vi "电源管理UI.vi"() -> ()   [LabVIEW 2016, in "PLC.lvlib"]
uses:
  PLC.lvlib
  <vilib>/Utility/miscctls.llb/LVPointTypeDef.ctl
  API/CodCr/CodCr.lvlib
panel:
  out "CODCr空闲时间":dbl caption="空闲时间:"
  out "总磷总氮空闲时间":dbl caption="空闲时间:"
  out "营养盐空闲时间":dbl caption="空闲时间:"
  out "CODMn空闲时间":dbl caption="空闲时间:"
  out "多参数空闲时间":dbl caption="空闲时间:"
  in  "CODCr电源":bool
  in  "总磷总氮电源":bool
  in  "营养盐电源":bool
  in  "CODMn电源":bool
  in  "多参数电源":bool
  # "说明：\n系统模式处于维护模式时，仪器电源自动打开；\n系统模式处于常规模式/质控模式/应急模式下，周期启动时，仪器电源打开，仪器空闲超过3600秒自动断电；"
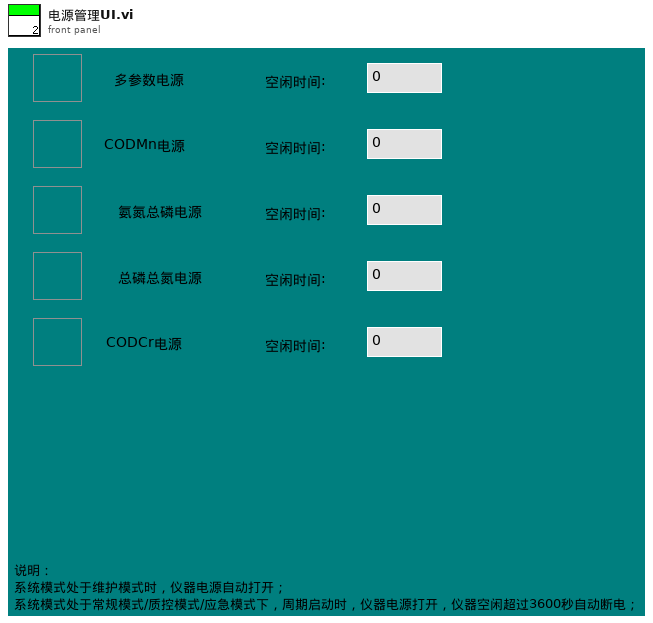
[diagram p1: front panel]
types:
  T1 = typedef "LVPointTypeDef.ctl" = cluster{"Horizontal":i16, "Vertical":i16}
  T2 = enum16{"空闲", "水样测试", "标样核查", "零点核查", "跨度核查", "空白测试", "平行样测试", "加标回收", "空白校准", "标样校准", "初始化（清洗）"}
  T3 = cluster{"系统时间":timestamp, "工作状态":u16, "测量模式":u16, "告警代码":enum16{"无告警", "缺试剂告警", "缺水样告警", "缺蒸馏水告警", "缺标液告警", "仪表漏液告警", "标定异常告警", "超量程告警", "加热异常", "低试剂预警", "超上限告警", "超下限告警", "仪表内部其他异常", "滴定异常告警", "电极异常告警", "量程切换告警", "参数设置告警", "PH电极电位异常", "电导率电极异常", "浊度光度异常", "溶解氧电极异常", "溶解氧光强异常", "温度异常告警", "PH异常告警", "溶解氧异常告警", "电导率异常告警", "浊度异常告警", "叶绿素异常告警", "藻密度异常告警", "蓝绿藻异常告警", "ORP异常告警", "氨氮异常告警", "清洁刷异常告警", "SD卡异常告警", "蓝牙异常告警", "Wifi异常告警", "流程异常告警"}, "故障代码":enum16{"无故障", "电机故障", "温度故障", "通讯故障", "滴定故障"}, "日志代码":u16, "软件版本":string}
  T4 = cluster{"系统时间":timestamp, "工作状态":enum16{"空闲", "水样测试", "标样核查", "零点核查", "跨度核查", "空白测试", "平行样测试", "加标回收", "空白校准", "标样校准", "初始化（清洗）"}, "测量模式":enum16{"待机", "连续模式", "周期模式", "定点模式", "受控模式", "手动模式"}, "告警代码":enum16{"无告警", "缺试剂告警", "缺水样告警", "缺蒸馏水告警", "缺标液告警", "仪表漏液告警", "标定异常告警", "超量程告警", "加热异常", "低试剂预警", "超上限告警", "超下限告警", "仪表内部其他异常", "滴定异常告警", "电极异常告警", "量程切换告警", "参数设置告警", "PH电极电位异常", "电导率电极异常", "浊度光度异常", "溶解氧电极异常", "溶解氧光强异常", "温度异常告警", "PH异常告警", "溶解氧异常告警", "电导率异常告警", "浊度异常告警", "叶绿素异常告警", "藻密度异常告警", "蓝绿藻异常告警", "ORP异常告警", "氨氮异常告警", "清洁刷异常告警", "SD卡异常告警", "蓝牙异常告警", "Wifi异常告警", "流程异常告警"}, "故障代码":enum16{"无故障", "电机故障", "温度故障", "通讯故障", "滴定故障"}, "日志代码":u16, "软件版本":u16, "F0":sgl, "F1":sgl, "F2":sgl, "F3":sgl, "T":sgl, "H":sgl, "id":u16, "flowid":u16, "量程":u16, "总磷控温温度1":sgl, "营养盐控温温度2":sgl, "ADC":sgl}
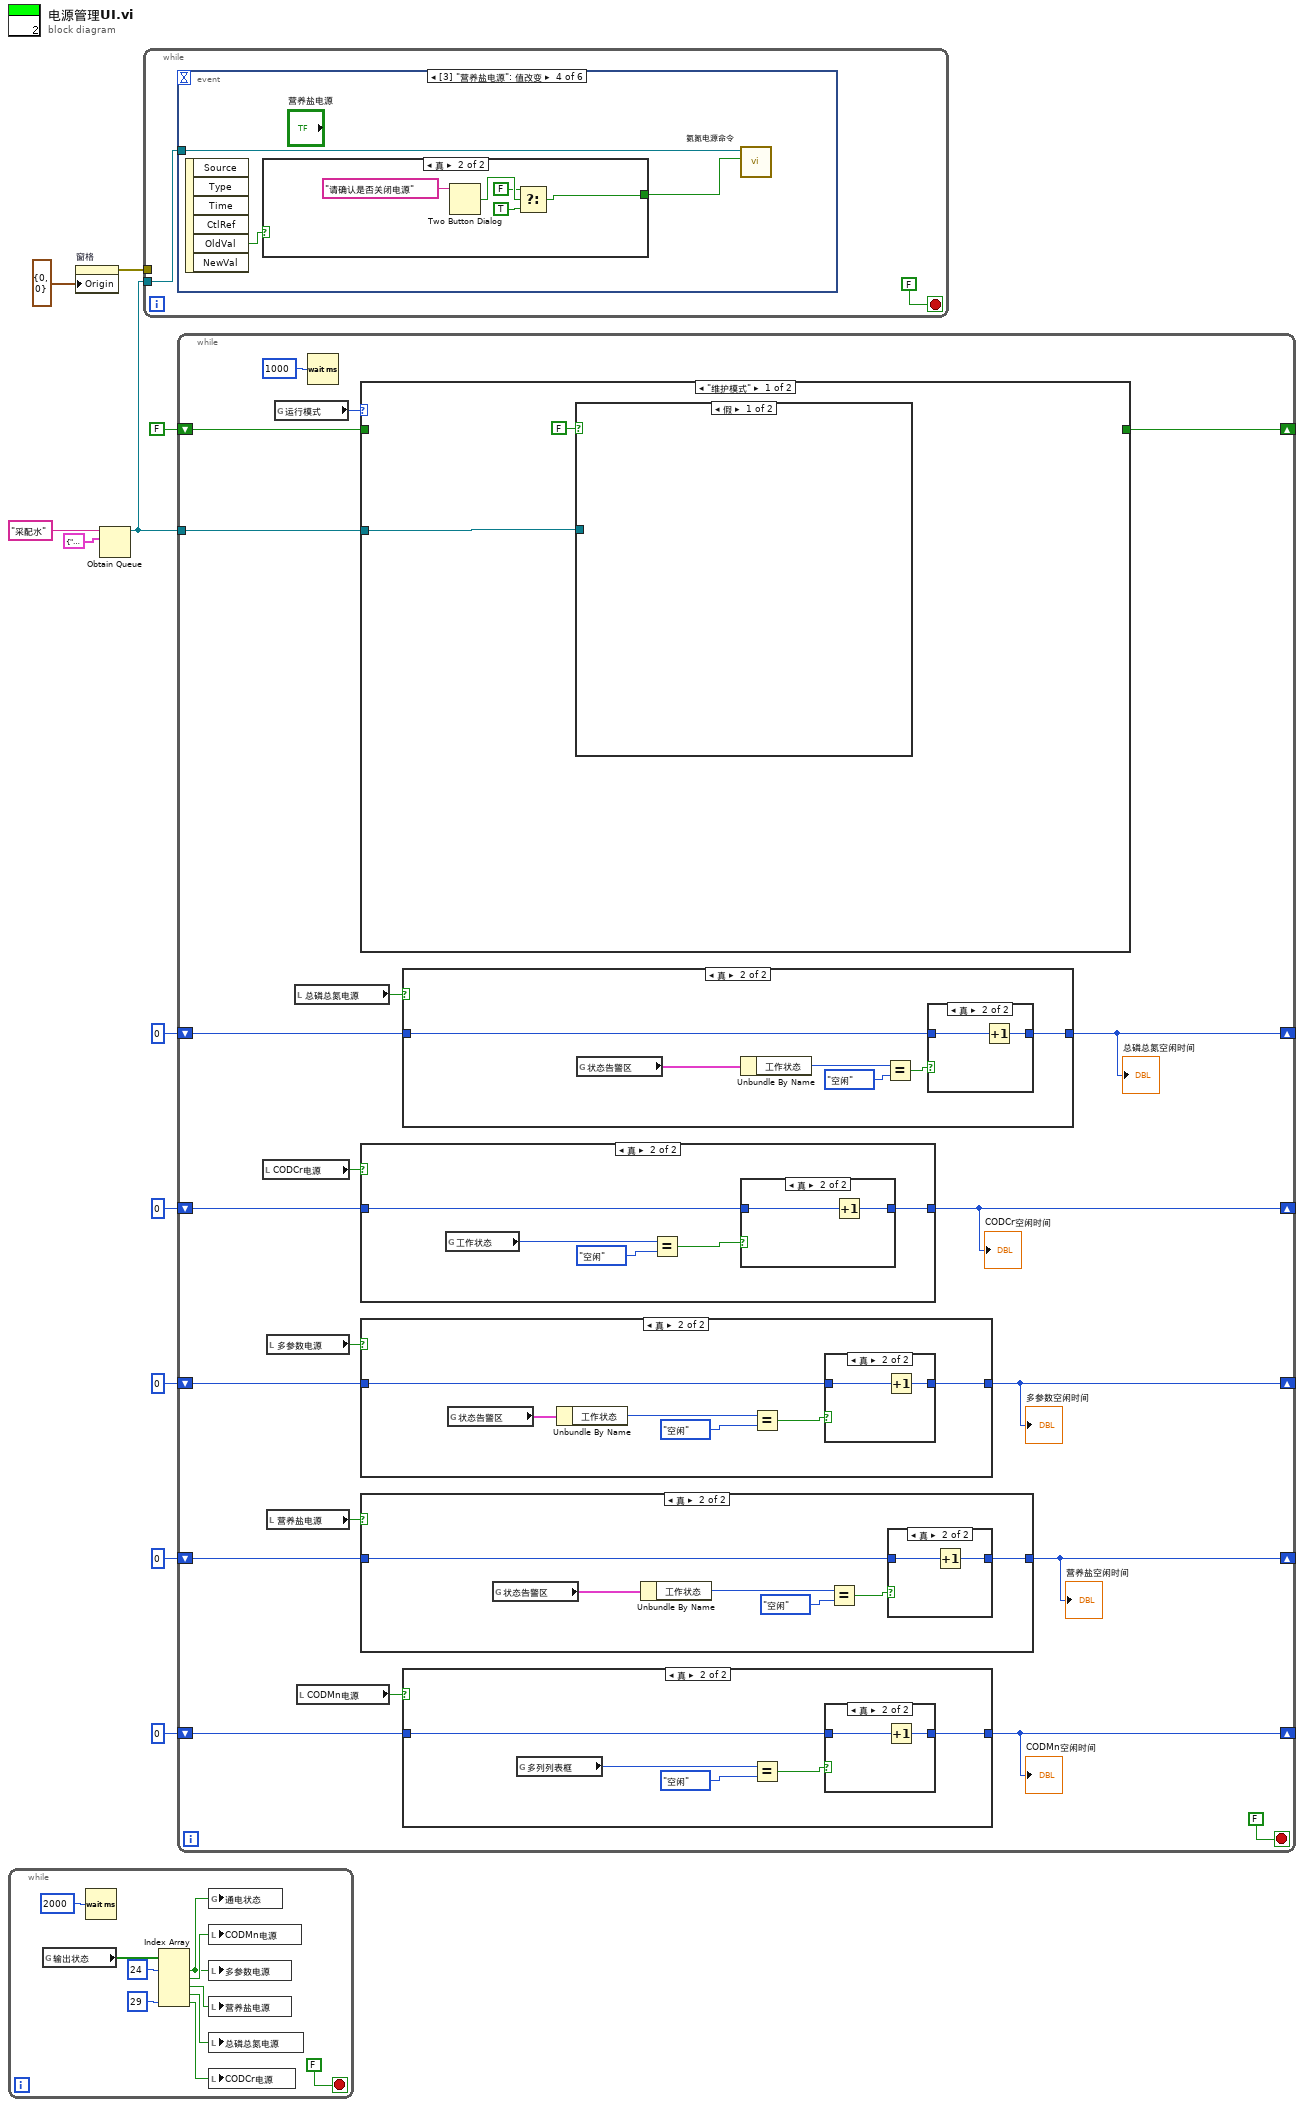
[diagram p0: block diagram]
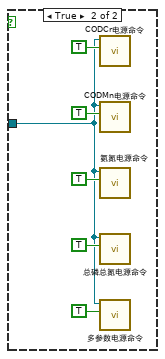
[diagram p2: hidden frame]
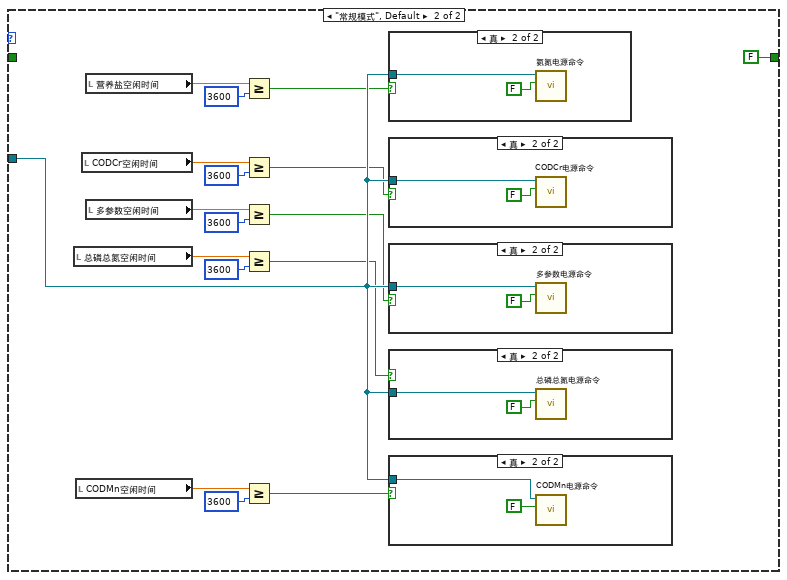
[diagram p3: hidden frame]
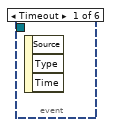
[diagram p19: hidden frame]
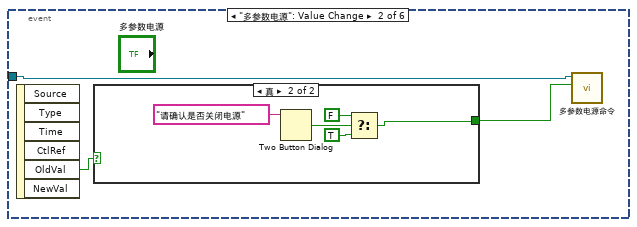
[diagram p20: hidden frame]
diagram:
  n1 = while {
    stop <- FALSE stop-if-true
    n2 = global read "采配水全局变量.vi" "输出状态"() -> (w19:bool[])
    n3 = Wait (ms)(milliseconds to wait=u32 2000 ("等待时间（毫秒）")) -> ()  [unwired: 1 out]
    n4 = Index Array(array=w19, index #1=24 ("索引"), index #5=29 ("索引")) -> (element #1=w14:bool, element #2=w17:bool, element #3=w16:bool, element #4=w15:bool, element #5=w13:bool)  [unwired: 3 in]
    n5 = global write "多参数全局变量.vi" "通电状态"(w14) -> ()
    n6 = local write "CODMn电源"(w17) -> ()
    n7 = local write "多参数电源"(w14) -> ()
    n8 = local write "营养盐电源"(w16) -> ()
    n9 = local write "总磷总氮电源"(w15) -> ()
    n10 = local write "CODCr电源"(w13) -> ()
  }
  n11 = property on="窗格" class="Pane"("Origin"=T1 {"Horizontal"=0, "Vertical"=0} ("原点")) -> (error out=w8:errorcluster)  [unwired: 2 in, 1 out]
  n12 = Obtain Queue(name (unnamed)="采配水" ("名称（未命名）"), element data type=cluster{"命令":string, "数据":variant} {"命令"="", "数据"=variant}) -> (queue out=w7:refnum<queue>)  [unwired: 3 in, 2 out]
  n13 = while {
    tunnel: w7 -> [w22]
    tunnel: w8 -> [_]
    stop <- FALSE stop-if-true
    n14 = event shown="[3] \"营养盐电源\": 值改变" {
      selector: _ -> [_ _ _ _ _ _]
      dyn-events: _ -> [_ _ _ _ _ _]
      timeout: _ -> [_ _ _ _ _ _]
      tunnel: w22 -> [_ w26 w35 w44 w53 w62]
      event Timeout {
        n15 = event-data() -> ()  [unwired: 1 in, 3 out]
      }
      event "多参数电源": Value Change {
        n16 = event-data() -> ("OldVal"=w25:bool)  [unwired: 1 in, 5 out]
        n17 = case shown="真" w25 {
          tunnel: [TRUE ("T button?") w28] -> w24
          frame False {
          }
          frame True {
            n18 = Two Button Dialog(message="请确认是否关闭电源" ("消息")) -> (T button?=w31:bool)  [unwired: 2 in]
            n19 = Select(t=FALSE, s=w31, f=TRUE ("T button?")) -> (s? t:f=w28:bool)
          }
        }
        n20 = call "多参数电源命令.vi"("通电/断电"=w24, "队列"=w26) -> ()  [unwired: 9 in, 1 out]
      }
      event "CODMn电源": Value Change {
        n21 = event-data() -> ("OldVal"=w34:bool)  [unwired: 1 in, 5 out]
        n22 = case shown="真" w34 {
          tunnel: [TRUE ("T button?") w37] -> w33
          frame False {
          }
          frame True {
            n23 = Two Button Dialog(message="请确认是否关闭电源" ("消息")) -> (T button?=w40:bool)  [unwired: 2 in]
            n24 = Select(t=FALSE, s=w40, f=TRUE ("T button?")) -> (s? t:f=w37:bool)
          }
        }
        n25 = call "CODMn电源命令.vi"("通电/断电"=w33, "队列"=w35) -> ()  [unwired: 9 in, 1 out]
      }
      event "营养盐电源": Value Change {
        n26 = event-data() -> ("OldVal"=w43:bool)  [unwired: 1 in, 5 out]
        n27 = case shown="真" w43 {
          tunnel: [TRUE ("T button?") w46] -> w42
          frame False {
          }
          frame True {
            n28 = Two Button Dialog(message="请确认是否关闭电源" ("消息")) -> (T button?=w49:bool)  [unwired: 2 in]
            n29 = Select(t=FALSE, s=w49, f=TRUE ("T button?")) -> (s? t:f=w46:bool)
          }
        }
        n30 = call "氨氮电源命令.vi"("通电/断电"=w42, "队列"=w44) -> ()  [unwired: 9 in, 1 out]
      }
      event "总磷总氮电源": Value Change {
        n31 = event-data() -> ("OldVal"=w52:bool)  [unwired: 1 in, 5 out]
        n32 = case shown="真" w52 {
          tunnel: [TRUE ("T button?") w55] -> w51
          frame False {
          }
          frame True {
            n33 = Two Button Dialog(message="请确认是否关闭电源" ("消息")) -> (T button?=w58:bool)  [unwired: 2 in]
            n34 = Select(t=FALSE, s=w58, f=TRUE ("T button?")) -> (s? t:f=w55:bool)
          }
        }
        n35 = call "总磷总氮电源命令.vi"("通电/断电"=w51, "队列"=w53) -> ()  [unwired: 9 in, 1 out]
      }
      event "CODCr电源": Value Change {
        n36 = event-data() -> ("OldVal"=w61:bool)  [unwired: 1 in, 5 out]
        n37 = case shown="真" w61 {
          tunnel: [TRUE ("T button?") w64] -> w60
          frame False {
          }
          frame True {
            n38 = Two Button Dialog(message="请确认是否关闭电源" ("消息")) -> (T button?=w67:bool)  [unwired: 2 in]
            n39 = Select(t=FALSE, s=w67, f=TRUE ("T button?")) -> (s? t:f=w64:bool)
          }
        }
        n40 = call "CODCr电源命令.vi"("通电/断电"=w60, "队列"=w62) -> ()  [unwired: 9 in, 1 out]
      }
    }
  }
  n41 = while {
    tunnel: w7 -> [w72]
    shift-right: [w73] -> _
    shift-left: u32 0 ("等待时间（毫秒）") -> [w86]
    shift-right: [w77] -> _
    shift-left: u32 0 ("等待时间（毫秒）") -> [w84]
    shift-right: [w75] -> _
    shift-left: u32 0 ("等待时间（毫秒）") -> [w80]
    shift-right: [w76] -> _
    shift-left: u32 0 ("等待时间（毫秒）") -> [w81]
    shift-right: [w74] -> _
    shift-left: u32 0 ("等待时间（毫秒）") -> [w79]
    shift-right: [w69] -> _
    shift-left: FALSE -> [w70]
    stop <- FALSE stop-if-true
    n42 = local read "CODCr电源"() -> (w78:bool)
    n43 = local read "多参数电源"() -> (w82:bool)
    n44 = local read "营养盐电源"() -> (w87:bool)
    n45 = global read "系统变量.vi" "运行模式"() -> (w71:enum16{"维护模式", "常规模式", "应急模式", "质控模式"})
    n46 = local read "总磷总氮电源"() -> (w83:bool)
    n47 = local read "CODMn电源"() -> (w85:bool)
    n48 = Wait (ms)(milliseconds to wait=u32 1000 ("等待时间（毫秒）")) -> ()  [unwired: 1 out]
    n49 = case shown="\"维护模式\"" w71 {
      tunnel: w72 -> [w91 w114]
      tunnel: w70 -> [_ _]
      tunnel: [_ FALSE] -> w69
      frame "维护模式" {
        n50 = case shown="假" FALSE {
          tunnel: w91 -> [_ w92]
          frame False {
          }
          frame True {
            n51 = call "CODCr电源命令.vi"("通电/断电"=TRUE, "队列"=w92) -> ()  [unwired: 9 in, 1 out]
            n52 = call "CODMn电源命令.vi"("通电/断电"=TRUE, "队列"=w92) -> ()  [unwired: 9 in, 1 out]
            n53 = call "氨氮电源命令.vi"("通电/断电"=TRUE, "队列"=w92) -> ()  [unwired: 9 in, 1 out]
            n54 = call "总磷总氮电源命令.vi"("通电/断电"=TRUE, "队列"=w92) -> ()  [unwired: 9 in, 1 out]
            n55 = call "多参数电源命令.vi"("通电/断电"=TRUE, "队列"=w92) -> ()  [unwired: 9 in, 1 out]
          }
        }
      }
      frame "常规模式", Default {
        n56 = local read "总磷总氮空闲时间"() -> (w99:dbl)
        n57 = local read "CODMn空闲时间"() -> (w102:dbl)
        n58 = local read "CODCr空闲时间"() -> (w109:dbl)
        n59 = local read "营养盐空闲时间"() -> (w105:dbl)
        n60 = local read "多参数空闲时间"() -> (w108:dbl)
        n61 = Greater Or Equal?(x=w105, y=u32 3600) -> (x >= y?=w107:bool)
        n62 = Greater Or Equal?(x=w109, y=u32 3600) -> (x >= y?=w111:bool)
        n63 = Greater Or Equal?(x=w108, y=u32 3600) -> (x >= y?=w113:bool)
        n64 = Greater Or Equal?(x=w99, y=u32 3600) -> (x >= y?=w101:bool)
        n65 = Greater Or Equal?(x=w102, y=u32 3600) -> (x >= y?=w104:bool)
        n66 = case shown="真" w107 {
          tunnel: w114 -> [_ w120]
          frame False {
          }
          frame True {
            n67 = call "氨氮电源命令.vi"("通电/断电"=FALSE, "队列"=w120) -> ()  [unwired: 9 in, 1 out]
          }
        }
        n68 = case shown="真" w111 {
          tunnel: w114 -> [_ w122]
          frame False {
          }
          frame True {
            n69 = call "CODCr电源命令.vi"("通电/断电"=FALSE, "队列"=w122) -> ()  [unwired: 9 in, 1 out]
          }
        }
        n70 = case shown="真" w113 {
          tunnel: w114 -> [_ w124]
          frame False {
          }
          frame True {
            n71 = call "多参数电源命令.vi"("通电/断电"=FALSE, "队列"=w124) -> ()  [unwired: 9 in, 1 out]
          }
        }
        n72 = case shown="真" w101 {
          tunnel: w114 -> [_ w116]
          frame False {
          }
          frame True {
            n73 = call "总磷总氮电源命令.vi"("通电/断电"=FALSE, "队列"=w116) -> ()  [unwired: 9 in, 1 out]
          }
        }
        n74 = case shown="真" w104 {
          tunnel: w114 -> [_ w118]
          frame False {
          }
          frame True {
            n75 = call "CODMn电源命令.vi"("通电/断电"=FALSE, "队列"=w118) -> ()  [unwired: 9 in, 1 out]
          }
        }
      }
    }
    n76 = case shown="真" w78 {
      tunnel: w79 -> [_ w129]
      tunnel: [_ w126] -> w74
      frame False {
      }
      frame True {
        n77 = global read "CODcr全局变量.vi" "工作状态"() -> (w125:T2)
        n78 = Equal?(x=w125, y=T2."空闲" ("工作状态")) -> (x = y?=w127:bool)
        n79 = case shown="真" w127 {
          tunnel: w129 -> [_ w131]
          tunnel: [_ w130] -> w126
          frame False {
          }
          frame True {
            n80 = Increment(x=w131) -> (x+1=w130:u32)
          }
        }
      }
    }
    "CODCr空闲时间" <- w74
    n81 = case shown="真" w82 {
      tunnel: w80 -> [_ w137]
      tunnel: [_ w134] -> w75
      frame False {
      }
      frame True {
        n82 = global read "多参数全局变量.vi" "状态告警区"() -> (w133:T3)
        n83 = Unbundle By Name(w133) -> ("工作状态"=w132:u16)
        n84 = Equal?(x=w132, y=T2."空闲" ("工作状态")) -> (x = y?=w135:bool)
        n85 = case shown="真" w135 {
          tunnel: w137 -> [_ w139]
          tunnel: [_ w138] -> w134
          frame False {
          }
          frame True {
            n86 = Increment(x=w139) -> (x+1=w138:u32)
          }
        }
      }
    }
    "多参数空闲时间" <- w75
    n87 = case shown="真" w87 {
      tunnel: w86 -> [_ w160]
      tunnel: [_ w156] -> w73
      frame False {
      }
      frame True {
        n88 = global read "VAR总磷氨氮全局变量.vi" "状态告警区"() -> (w155:T4)
        n89 = Unbundle By Name(w155) -> ("工作状态"=w159:T2)
        n90 = Equal?(x=w159, y=T2."空闲" ("工作状态")) -> (x = y?=w157:bool)
        n91 = case shown="真" w157 {
          tunnel: w160 -> [_ w162]
          tunnel: [_ w161] -> w156
          frame False {
          }
          frame True {
            n92 = Increment(x=w162) -> (x+1=w161:u32)
          }
        }
      }
    }
    "营养盐空闲时间" <- w73
    n93 = case shown="真" w83 {
      tunnel: w81 -> [_ w145]
      tunnel: [_ w142] -> w76
      frame False {
      }
      frame True {
        n94 = global read "VAR总磷氨氮全局变量.vi" "状态告警区"() -> (w141:T4)
        n95 = Unbundle By Name(w141) -> ("工作状态"=w140:T2)
        n96 = Equal?(x=w140, y=T2."空闲" ("工作状态")) -> (x = y?=w143:bool)
        n97 = case shown="真" w143 {
          tunnel: w145 -> [_ w147]
          tunnel: [_ w146] -> w142
          frame False {
          }
          frame True {
            n98 = Increment(x=w147) -> (x+1=w146:u32)
          }
        }
      }
    }
    "总磷总氮空闲时间" <- w76
    n99 = case shown="真" w85 {
      tunnel: w84 -> [_ w152]
      tunnel: [_ w149] -> w77
      frame False {
      }
      frame True {
        n100 = global read "运行时序全局变量.vi" "多列列表框"() -> (w148:i32)
        n101 = Equal?(x=w148, y=T2."空闲" ("工作状态")) -> (x = y?=w150:bool)
        n102 = case shown="真" w150 {
          tunnel: w152 -> [_ w154]
          tunnel: [_ w153] -> w149
          frame False {
          }
          frame True {
            n103 = Increment(x=w154) -> (x+1=w153:u32)
          }
        }
      }
    }
    "CODMn空闲时间" <- w77
  }
